vi "peredatchikdanden.vi"() -> ()   [LabVIEW 2020]
panel:
  in  "2 Зн-е температуры":dbl(knob) scale=0.0..90.0
  in  "1 Зн-е температуры":dbl(knob) scale=0.0..90.0
  in  "порта отправления":u16=50000
  in  "Адрес получателя":string="127.0.0.1"
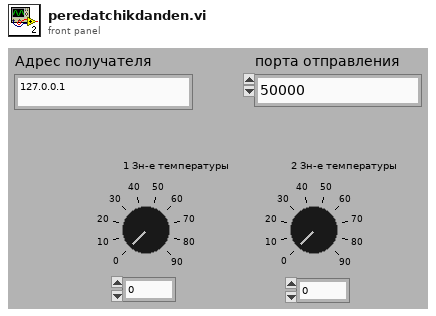
[diagram p1: front panel]
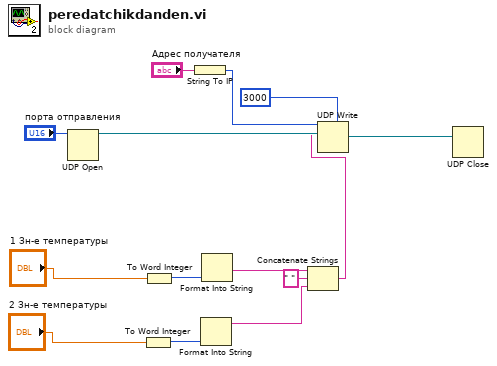
[diagram p0: block diagram]
diagram:
  n1 = UDP Open(11:"порта отправления") -> (port=w12:refnum<k16>)  [unwired: 4 in, 2 out]
  n2 = To Word Integer(number="2 Зн-е температуры") -> (16bit integer=w2:i16)
  n3 = To Word Integer(number="1 Зн-е температуры") -> (16bit integer=w7:i16)
  n4 = String To IP(1:"Адрес получателя") -> (0:w9:u32)
  n5 = Format Into String(w2) -> (resulting string=w1:string)  [unwired: 3 in, 1 out]
  n6 = Format Into String(w7) -> (resulting string=w5:string)  [unwired: 3 in, 1 out]
  n7 = Concatenate Strings(w5, " " ("string"), w1) -> (w6:string)
  n8 = UDP Write(address=w9, port or service name=u16 3000 ("port"), connection ID=w12, data in=w6) -> (3:w11:refnum<k16>)  [unwired: 2 in, 1 out]
  n9 = UDP Close(connection ID=w11) -> ()  [unwired: 1 in, 2 out]
